vi "WDT Get Final Time Value DBL.vi"(7 "open interval? (T)":bool=TRUE, 8 "error in (no error)":errorcluster, 11 "waveform in":waveform(dbl)) -> (0 "error out":errorcluster, 2 "tf":timestamp, 3 "waveform out":waveform(dbl))   [LabVIEW 2020]
doc: "Returns the ending time value of <B>waveform in</B>. The formula used is xf = x0 + duration of <B>waveform in</B>. Wire data to the <B>waveform in</B> input to determine the polymorphic instance to use or manually select the instance."
panel:
  in  "Waveform ERROR":waveform(dbl)={"t0"=timestamp(0 s since 1904-01-01), "dt"=0.0, "Y"=[]}
  # "open"
  # "closed"
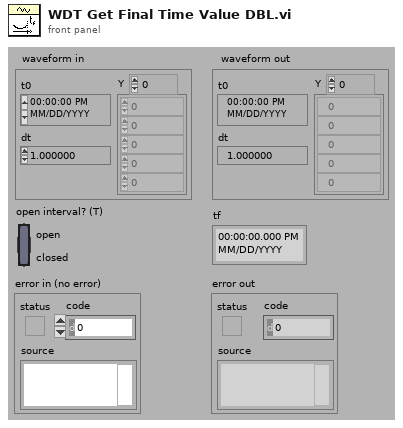
[diagram p1: front panel]
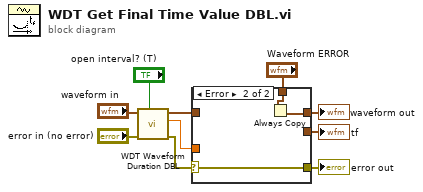
[diagram p0: block diagram]
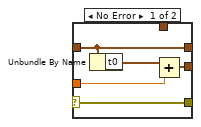
[diagram p2: hidden frame]
diagram:
  n1 = call "WDT Waveform Duration DBL.vi"("open interval? (T)"="open interval? (T)", "error in (no error)"="error in (no error)", "waveform in"="waveform in") -> ("error out"=w3:errorcluster, "duration"=w9:dbl, "waveform out"=w4:waveform(dbl))  [unwired: 6 in]
  n2 = case shown="Error" w3 {
    selector: w3 -> [w12 w17]
    tunnel: w4 -> [w13 _]
    tunnel: [w13 w16] -> w7
    tunnel: w9 -> [w15 _]
    tunnel: [w14 _] -> w8
    tunnel: "Waveform ERROR" -> [_ w18]
    tunnel: [w12 w17] -> w2
    frame No Error {
      n3 = Unbundle By Name(w13) -> ("t0"=w11:timestamp)
      n4 = Add(x=w11, y=w15) -> (x+y=w14:timestamp)
    }
    frame Error {
      n5 = Always Copy(1:w18) -> (0:w16:waveform(dbl))
    }
  }
  "tf" <- w8
  "waveform out" <- w7
  "error out" <- w2
